vi "CleanUp.vi"(0 "object in":refnum<class "TDMSLogger_PowerScan.lvclass">, 5 "error in (no error)":errorcluster) -> (14 "object out":refnum<class "TDMSLogger_PowerScan.lvclass">, 19 "error out":errorcluster)   [LabVIEW 2023, in "TDMSLogger_PowerScan.lvclass"]
uses:
  TDMSLogger_PowerScan.lvclass
  TDMSLogger_PowerScan.lvclass/TDMSLogger_PowerScan.ctl
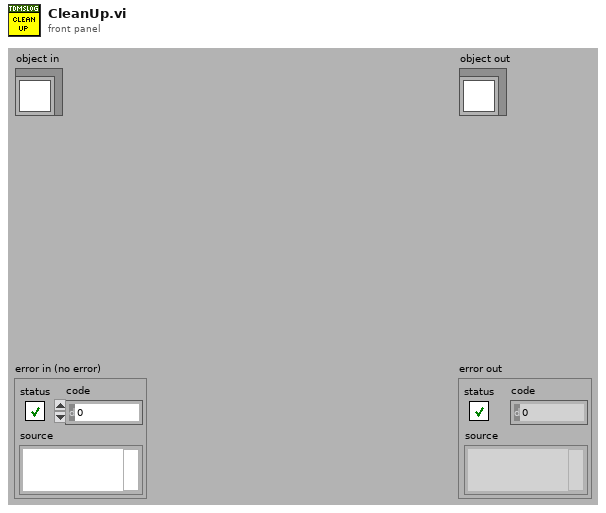
[diagram p1: front panel]
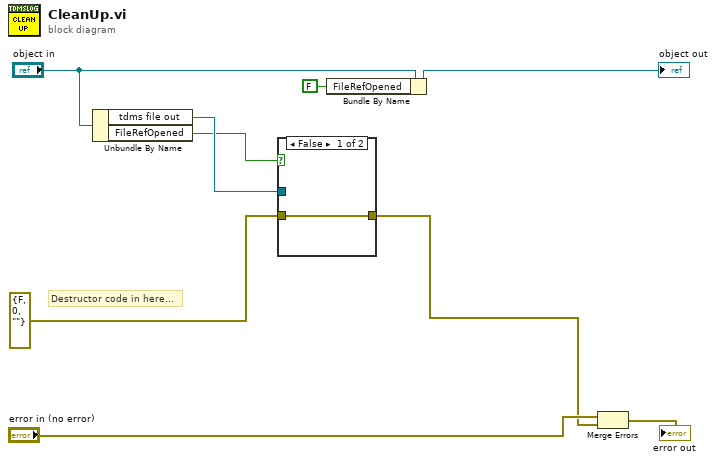
[diagram p0: block diagram]
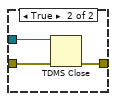
[diagram p2: hidden frame]
diagram:
  # "Destructor code in here..."
  n1 = Unbundle By Name("object in") -> ("tdms file out"=w6:refnum<k34>, "FileRefOpened"=w3:bool)
  n2 = case shown="False" w3 {
    tunnel: w6 -> [_ w13]
    tunnel: errorcluster {"status"=FALSE, "code"=0, "source"=""} ("error in (no error)") -> [w10 w12]
    tunnel: [w10 w11] -> w4
    frame False {
    }
    frame True {
      n3 = TDMS Close(8:w12, 11:w13) -> (0:w11:errorcluster)  [unwired: 1 out]
    }
  }
  n4 = Bundle By Name(cluster="object in", "FileRefOpened"=FALSE) -> (→"object out":refnum<class "TDMSLogger_PowerScan.lvclass">)
  n5 = Merge Errors("error in (no error)", w4) -> (→"error out":errorcluster)
